vi "Reset.vi"(8 "error in (no error)":errorcluster, 9 "Direction":T1, 10 "Position":T2, 11 "Mouse in":refnum<class "Mouse.lvclass">) -> (0 "error out":errorcluster, 3 "Mouse out":refnum<class "Mouse.lvclass">)   [LabVIEW 2020, in "Maze.lvlib" / "Mouse.lvclass"]
uses:
  Mouse.lvclass
  Position.ctl
  Direction.ctl
  Mouse.lvclass/Mouse.ctl
  Maze.lvlib
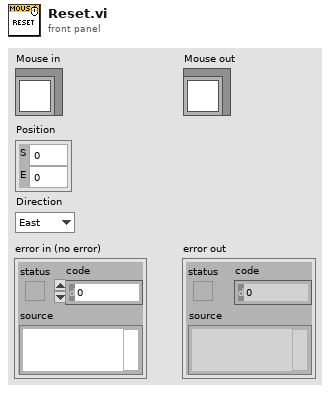
[diagram p1: front panel]
types:
  T1 = typedef "Maze.lvlib/Direction.ctl" = enum8{"East", "North", "West", "South"}
  T2 = typedef "Maze.lvlib/Position.ctl" = cluster{"S":i32, "E":i32}
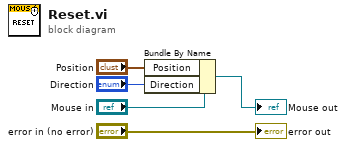
[diagram p0: block diagram]
diagram:
  n1 = Bundle By Name(cluster="Mouse in", "Position"="Position", "Direction"="Direction") -> (→"Mouse out":refnum<class "Mouse.lvclass">)
  "error out" <- "error in (no error)"
